vi "MediaCH.vi"(0 "input cluster":T1, 13 "Data":waveform(dbl)[](array[waveform])) -> (4 "Mitja CH1":dbl format="%0.2f", 6 "Mitja CH2":dbl format="%0.2f", 8 "Mitja CH3":dbl format="%0.2f", 10 "Mitja CH4":dbl format="%0.2f")   [LabVIEW 2014]
uses:
  <vilib>/Analysis/baseanly.llb/Mean (DBL).vi
  <vilib>/Waveform/WDTOps.llb/WDT Index Channel DBL.vi
  <vilib>/Analysis/NI_AALBase.lvlib
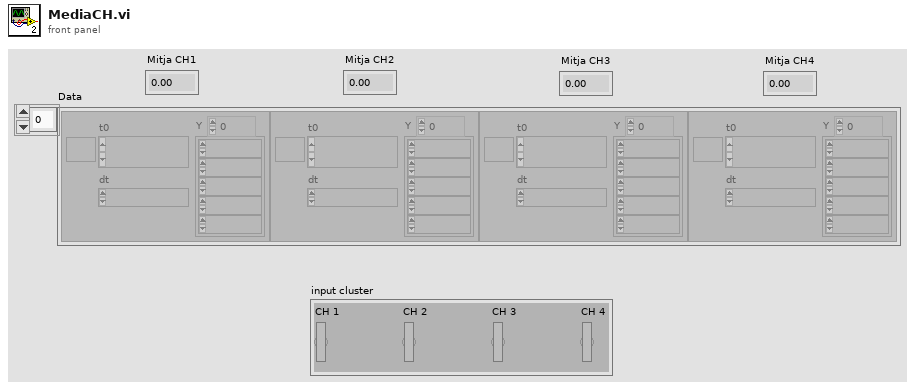
[diagram p1: front panel]
types:
  T1 = cluster{"CH 1":bool, "CH 2":bool, "CH 3":bool, "CH 4":bool}
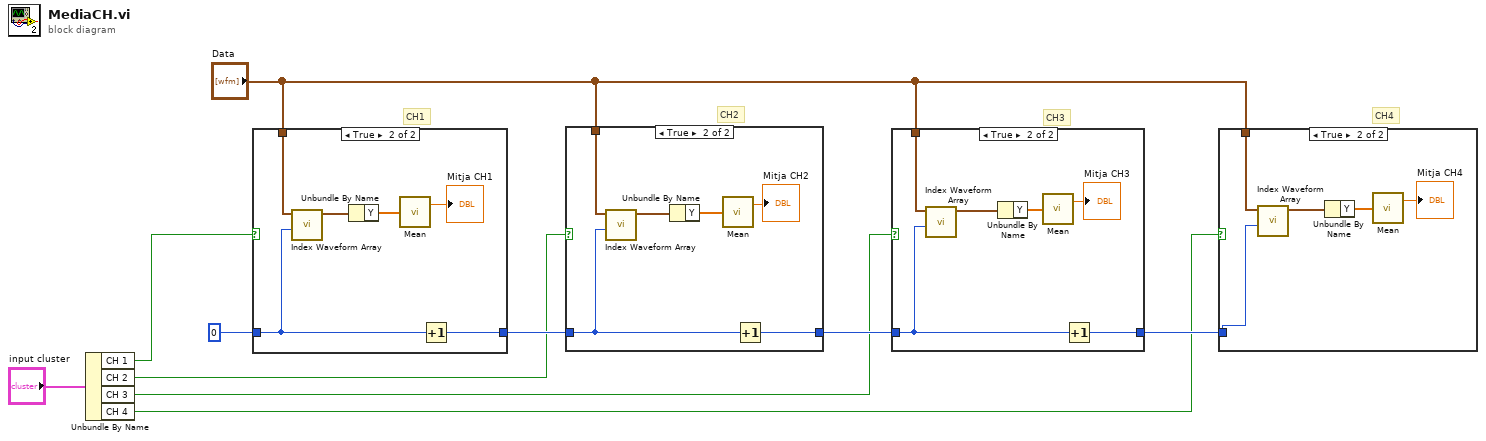
[diagram p0: block diagram]
diagram:
  # "CH4"
  # "CH3"
  # "CH2"
  # "CH1"
  n1 = Unbundle By Name("input cluster") -> ("CH 1"=w5:bool, "CH 2"=w4:bool, "CH 3"=w3:bool, "CH 4"=w2:bool)
  n2 = case shown="True" w5 {
    tunnel: 0 -> [w11 w16]
    tunnel: [w11 w15] -> w9
    tunnel: "Data" -> [_ w14]
    frame False {
    }
    frame True {
      n3 = call-poly <vilib>:"Index Waveform Array.vi"("index"=w16, "waveform array"=w14) -> ("waveform"=w13:waveform(dbl))  [unwired: 8 in, 1 out]
      n4 = Unbundle By Name(w13) -> ("Y"=w12:dbl[])
      n5 = call-poly <vilib>:"Mean.vi"("X"=w12) -> ("mean"=→"Mitja CH1":dbl)  [unwired: 1 out]
      n6 = Increment(x=w16) -> (x+1=w15:i32)
    }
  }
  n7 = case shown="True" w4 {
    tunnel: w9 -> [w18 w24]
    tunnel: [w18 w23] -> w8
    tunnel: "Data" -> [_ w22]
    frame False {
    }
    frame True {
      n8 = call-poly <vilib>:"Index Waveform Array.vi"("index"=w24, "waveform array"=w22) -> ("waveform"=w20:waveform(dbl))  [unwired: 8 in, 1 out]
      n9 = Unbundle By Name(w20) -> ("Y"=w19:dbl[])
      n10 = call-poly <vilib>:"Mean.vi"("X"=w19) -> ("mean"=→"Mitja CH2":dbl)  [unwired: 1 out]
      n11 = Increment(x=w24) -> (x+1=w23:i32)
    }
  }
  n12 = case shown="True" w3 {
    tunnel: w8 -> [w25 w31]
    tunnel: [w25 w30] -> w7
    tunnel: "Data" -> [_ w29]
    frame False {
    }
    frame True {
      n13 = call-poly <vilib>:"Index Waveform Array.vi"("index"=w31, "waveform array"=w29) -> ("waveform"=w27:waveform(dbl))  [unwired: 8 in, 1 out]
      n14 = Unbundle By Name(w27) -> ("Y"=w26:dbl[])
      n15 = call-poly <vilib>:"Mean.vi"("X"=w26) -> ("mean"=→"Mitja CH3":dbl)  [unwired: 1 out]
      n16 = Increment(x=w31) -> (x+1=w30:i32)
    }
  }
  n17 = case shown="True" w2 {
    tunnel: w7 -> [_ w36]
    tunnel: "Data" -> [_ w35]
    frame False {
    }
    frame True {
      n18 = call-poly <vilib>:"Index Waveform Array.vi"("index"=w36, "waveform array"=w35) -> ("waveform"=w33:waveform(dbl))  [unwired: 8 in, 1 out]
      n19 = Unbundle By Name(w33) -> ("Y"=w32:dbl[])
      n20 = call-poly <vilib>:"Mean.vi"("X"=w32) -> ("mean"=→"Mitja CH4":dbl)  [unwired: 1 out]
    }
  }
